vi "Update_Build_Instance.vi"(8 "error in (no error)":errorcluster, 10 "AppInstanceForBuild in":refnum<vi>, 11 "Build in":refnum<class "AB_Build.lvclass">) -> (0 "error out":errorcluster, 2 "AppInstanceForBuild out":refnum<vi>, 3 "Build out":refnum<class "AB_Build.lvclass">)   [LabVIEW 2020, in "AB_Build.lvclass"]
uses:
  <vilib>/AppBuilder/AB_Classes/Build/AB_Build.lvclass
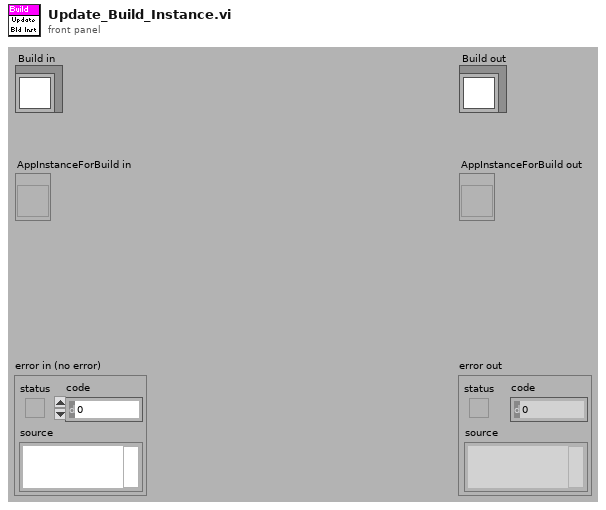
[diagram p1: front panel]
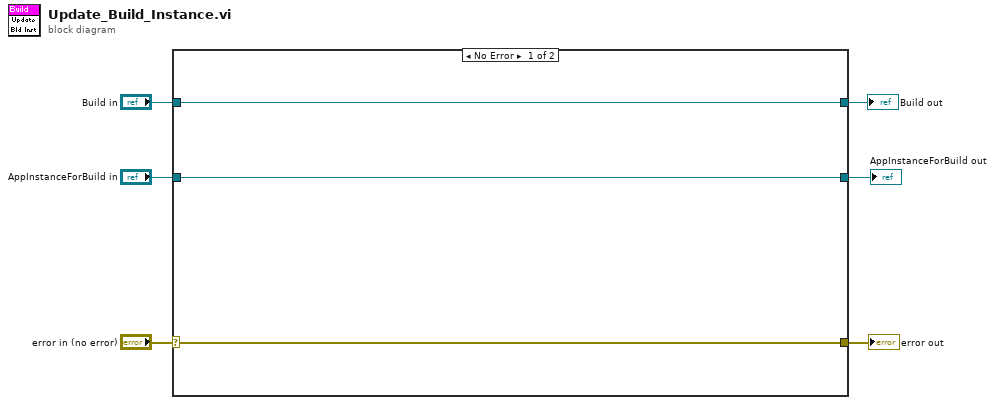
[diagram p0: block diagram]
diagram:
  n1 = case shown="No Error" "error in (no error)" {
    selector: "error in (no error)" -> [w9 w12]
    tunnel: [w9 w12] -> w5
    tunnel: [w8 w11] -> w3
    tunnel: "Build in" -> [w8 w11]
    tunnel: "AppInstanceForBuild in" -> [w7 w10]
    tunnel: [w7 w10] -> w1
    frame No Error {
    }
    frame Error {
    }
  }
  "error out" <- w5
  "Build out" <- w3
  "AppInstanceForBuild out" <- w1
